vi "檢測_找邊_VI.vi"(6 "Edge Options":T4={"Edge Polarity"=0, "Kernel Size"=3, "Width"=3, "Minimum Edge Strength"=10.0, "Interpolation Type"=enum."Bilinear Fixed", "Data Processing Method"=enum."Average"} {"Edge Polarity" items=["All Edges", "Rising Edges", "Falling Edges"]; "Minimum Edge Strength" format="%.2f"; "Width" step=2; "Kernel Size" step=2}, 7 "Scan Direction":u16(ring) items=["Left To Right", "Right To Left", "Top To Bottom", "Bottom To Top"], 8 "error in (no error)":errorcluster, 9 "Coordinate System":T1 {"Measurement System"."Axis Reference" items=["Direct", "Indirect"]; "Measurement System"."Angle (deg)" format="%.2f"; "Measurement System"."Origin"."Y" format="%.2f"; "Measurement System"."Origin"."X" format="%.2f"; "Reference System"."Axis Reference" items=["Direct", "Indirect"]; "Reference System"."Angle (deg)" format="%.2f"; "Reference System"."Origin"."Y" format="%.2f"; "Reference System"."Origin"."X" format="%.2f"}, 10 "ROI":T2, 11 "Image":T3) -> (0 "error out":errorcluster, 2 "Array":cluster{"X":sgl, "Y":sgl}[](array[cluster]), 3 "Image Out":T3)   [LabVIEW 2015]
uses:
  <vilib>/vision/Measure.llb/Edge Options.ctl
  <vilib>/vision/Measure.llb/Edge Polarity.ctl
  <vilib>/vision/Image Controls.llb/IMAQ Image.ctl
  <vilib>/vision/NI_Vision_Development_Module.lvlib
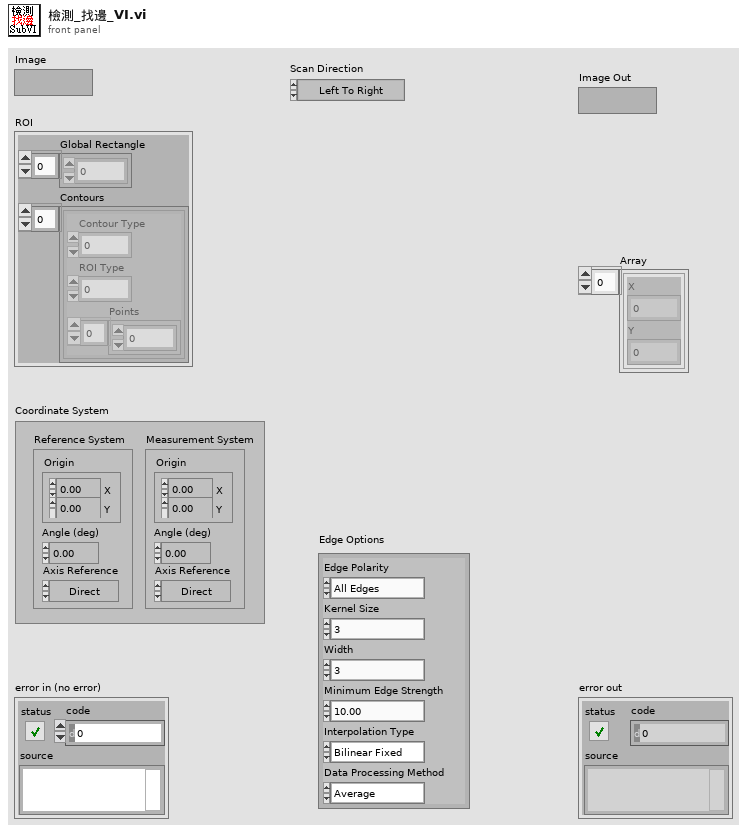
[diagram p1: front panel]
types:
  T1 = typedef "IMAQ Coordinate System" = cluster{"Reference System":cluster{"Origin":cluster{"X":sgl, "Y":sgl}, "Angle (deg)":sgl, "Axis Reference":u32}, "Measurement System":cluster{"Origin":cluster{"X":sgl, "Y":sgl}, "Angle (deg)":sgl, "Axis Reference":u32}}
  T2 = cluster{"Global Rectangle":i32[], "Contours":cluster{"Contour Type":u32, "ROI Type":u32, "Points":i32[]}[]}
  T3 = typedef "IMAQ Image.ctl" = refnum<image>
  T4 = typedef "Edge Options.ctl" = cluster{"Edge Polarity":T5, "Kernel Size":u32, "Width":u32, "Minimum Edge Strength":sgl, "Interpolation Type":enum32{"Zero Order", "Bilinear", "Quadratic", "Cubic", "Bilinear Fixed"}, "Data Processing Method":enum32{"Average", "Median"}}
  T5 = typedef "Edge Polarity.ctl" = u32
  T6 = cluster{"Origin":cluster{"X":sgl, "Y":sgl}, "Angle (deg)":sgl, "Axis Reference":u32}
  T7 = typedef "ROI Descriptor" = cluster{"Global Rectangle":i32[], "Contours":cluster{"ID":enum32{"External", "Internal"}, "Type":u32, "Coordinates":i32[]}[]}
  T8 = typedef "Edge New.ctl" = cluster{"Location (Pixel)":cluster{"X":sgl, "Y":sgl}, "Location (Real-World)":cluster{"X":sgl, "Y":sgl}, "Distance (Pixel)":dbl, "Distance (Real-World)":dbl, "Strength":dbl, "Noise":dbl, "Rising?":bool}
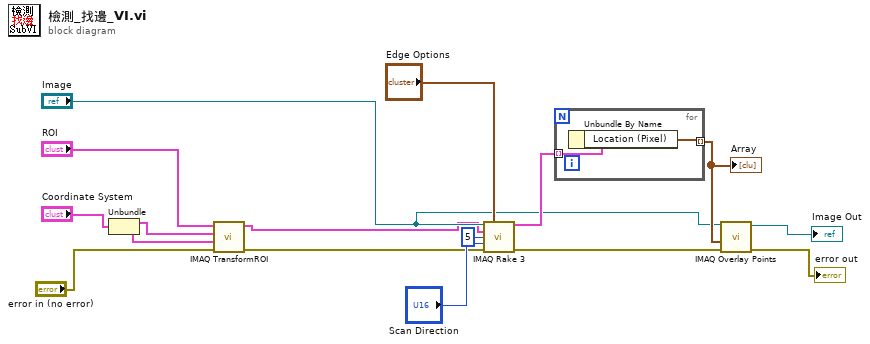
[diagram p0: block diagram]
diagram:
  n1 = Unbundle("Coordinate System") -> ("Reference System"=w3:T6, "Measurement System"=w2:T6)
  n2 = call "IMAQ TransformROI"("error in (no error)"="error in (no error)", "New Reference"=w2, "Base Reference"=w3, "ROI Descriptor"="ROI") -> ("error out"=w6:errorcluster, "ROI Descriptor out"=w1:T7)  [unwired: 6 in]
  n3 = call "IMAQ Rake 3"("Image"="Image", "Edge Options"="Edge Options", "ROI Descriptor"=w1, "Step Size"=u32 5, "Scan Direction"="Scan Direction", "error in (no error)"=w6) -> ("First Edges"=w14:T8[], "error out"=w15:errorcluster)  [unwired: 6 in, 2 out]
  n4 = for {
    tunnel: w14 -> [w18] mode=indexing
    tunnel: [w17] -> w13 mode=indexing
    n5 = Unbundle By Name(w18) -> ("Location (Pixel)"=w17:cluster{"X":sgl, "Y":sgl})
  }
  "Array" <- w13
  n6 = call "IMAQ Overlay Points"("error in (no error)"=w15, "Array of Points"=w13, "Image"="Image") -> ("error out"=→"error out":errorcluster, "Image Out"=→"Image Out":T3)  [unwired: 7 in]
